vi "BotSpeak.BaseCom.vi"(3 "Termination":string="\r\n", 5 "command":string="PING", 6 "Bot Settings in":T1) -> (0 "response":string="169.254.32.85", 2 "Bot Settings out":T1)   [LabVIEW 2012]
doc: "Protocol:\nLCD \"text to write\" 0,0 // start row, start col (0,0 default)\nBTN // replies with a 5 bit number bot PB1-PB5\nLED 64 // each bit corresponds to an LED\nAI 0 // replies with the value of A/D 0\nAO 2.5,1.34 // sets DAC 0 to 2.5 v and DAC 1 to 1.34 v\nDIO 3,1 // sets DIO 3 to HIGH\nDIO 3 // reads DIO 3 and returns state\nIP // returns IP Address\nTEMP // returns Temperature reading"
uses:
  <userlib>/BotSpeak/VIs/Direct/BotSpeak_Control.ctl
  <userlib>/BotSpeak/VIs/SubVIs/BotSpeak_Globals.vi
panel:
  # "GET DIO[DIO[1]}"
  # "to do:\n\n\nAbort does not work."
  # "use Address \"close\" to close the \nlast connection"
  # "blank means no reply"
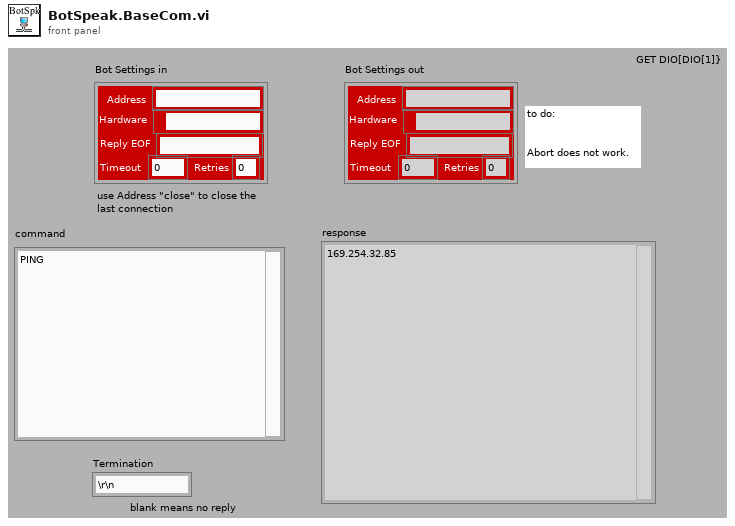
[diagram p1: front panel]
types:
  T1 = typedef "BotSpeak_Control.ctl" = cluster{"Address":string, "Reply EOF":string, "Hardware":path, "Retries":i8, "Timeout":i32}
  T2 = typedef "CommState.ctl" = cluster{"Bot Settings":T1, "Initialized":bool, "Talking":bool}
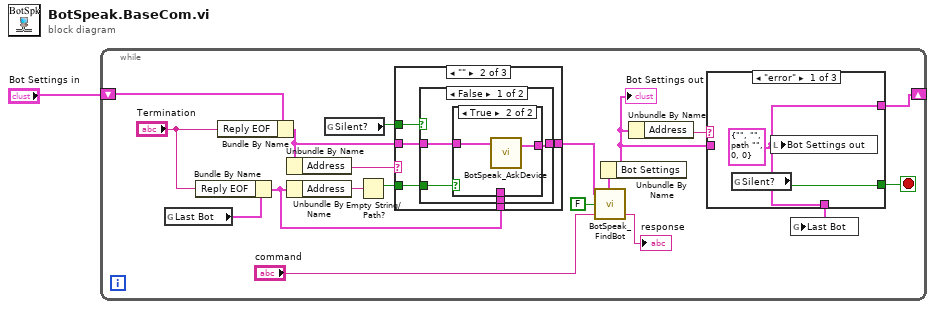
[diagram p0: block diagram]
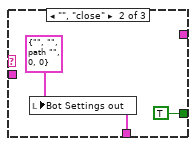
[diagram p2: hidden frame]
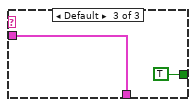
[diagram p3: hidden frame]
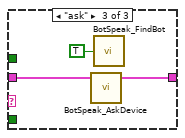
[diagram p7: hidden frame]
diagram:
  n1 = while {
    shift-right: [w3] -> _
    shift-left: "Bot Settings in" -> [w4]
    stop <- w5 stop-if-true
    n2 = global read "BotSpeak_Globals.vi" "Last Bot"() -> (w14:T1)
    n3 = Bundle By Name(cluster=w14, "Reply EOF"="Termination") -> (w12:T1)
    n4 = Bundle By Name(cluster=w4, "Reply EOF"="Termination") -> (w17:T1)
    n5 = Unbundle By Name(w17) -> ("Address"=w18:string)
    n6 = Unbundle By Name(w12) -> ("Address"=w20:string)
    n7 = global read "BotSpeak_Globals.vi" "Silent?"() -> (w2:bool)
    n8 = Empty String/Path?(string/path=w20) -> (empty?=w19:bool)
    n9 = case shown="\"\"" w18 {
      tunnel: [w27 w31 w42] -> w10
      tunnel: w17 -> [w27 w32 w43]
      tunnel: w19 -> [_ w30 _]
      tunnel: w12 -> [_ w29 _]
      tunnel: w2 -> [_ w28 _]
      frame Default {
      }
      frame "" {
        n10 = case shown="False" w28 {
          tunnel: w32 -> [w36 w40]
          tunnel: [w35 w40] -> w31
          tunnel: w30 -> [w34 _]
          tunnel: w29 -> [w33 _]
          frame False {
            n11 = case shown="True" w34 {
              tunnel: w36 -> [_ w39]
              tunnel: [w37 w38] -> w35
              tunnel: w33 -> [w37 _]
              frame False {
              }
              frame True {
                n12 = call <userlib>:"BotSpeak_AskDevice.vi"("Bot Settings"=w39) -> ("Bot Settings out"=w38:T1)  [unwired: 2 in]
              }
            }
          }
          frame True {
          }
        }
      }
      frame "ask" {
        n13 = call <userlib>:"BotSpeak_AskDevice.vi"("Bot Settings"=w43) -> ("Bot Settings out"=w42:T1)  [unwired: 2 in]
        n14 = call <userlib>:"BotSpeak_FindBot.vi"("Reset?"=TRUE) -> ()  [unwired: 2 in, 3 out]
      }
    }
    n15 = call <userlib>:"BotSpeak_FindBot.vi"("String To Send"="command", "Reset?"=FALSE, "Bot Settings"=w10) -> ("Reply"=→"response":string, "Connection"=w8:T2)  [unwired: 1 out]
    n16 = Unbundle By Name(w8) -> ("Bot Settings"=w7:T1)
    "Bot Settings out" <- w7
    n17 = Unbundle By Name(w7) -> ("Address"=w15:string)
    n18 = case shown="\"error\"" w15 {
      tunnel: w7 -> [_ _ w26]
      tunnel: [w22 w23 w26] -> w16
      tunnel: [w21 TRUE TRUE] -> w5
      tunnel: [w22 _ _] -> w3
      frame "error" {
        w22 = T1 {"Address"="", "Reply EOF"="", "Hardware"=path "", "Retries"=0, "Timeout"=0} ("Bot Settings Out")
        n19 = global read "BotSpeak_Globals.vi" "Silent?"() -> (w21:bool)
        n20 = local write "Bot Settings out"(w22) -> ()
      }
      frame "", "close" {
        w23 = T1 {"Address"="", "Reply EOF"="", "Hardware"=path "", "Retries"=0, "Timeout"=0} ("Bot Settings Out")
        n21 = local write "Bot Settings out"(w23) -> ()
      }
      frame Default {
      }
    }
    n22 = global write "BotSpeak_Globals.vi" "Last Bot"(w16) -> ()
  }
